vi "WPI_DashboardUpdate Table Values.vi"(11 "Data Values":variant[](array[variant])) -> ()   [LabVIEW 2025]
uses:
  <vilib>/Rock Robotics/WPI/Dashboard/WPI_DashboardLogging Global.vi
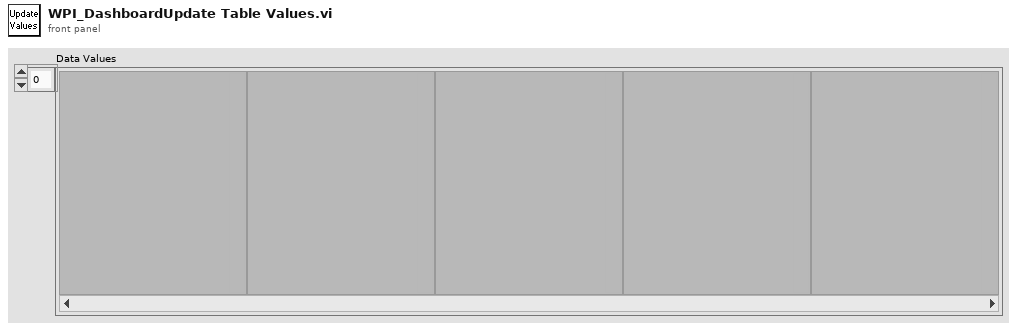
[diagram p1: front panel]
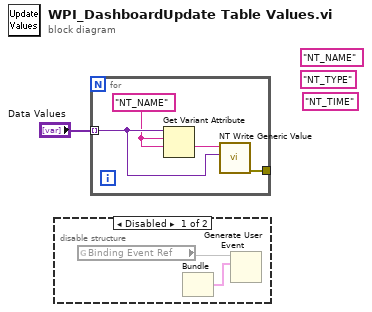
[diagram p0: block diagram]
diagram:
  (unwired) "NT_NAME" ("String")
  (unwired) "NT_TIME" ("String")
  (unwired) "NT_TYPE" ("String")
  n1 = disable-structure shown="Disabled" {
    frame Disabled {
      n2 = global read "WPI_DashboardLogging Global.vi" "Binding Event Ref"() -> (w3)
      n3 = Bundle() -> (w2:cluster{void, void, void})  [unwired: 4 in]
      n4 = Generate User Event(user event=w3, event data cluster=w2) -> ()  [unwired: 2 in, 2 out]
    }
    frame Enabled {
    }
  }
  n5 = for {
    tunnel: "Data Values" -> [w7] mode=indexing
    tunnel: [w4] -> _
    w5 = "NT_NAME" ("String")
    n6 = Get Variant Attribute(Variant=w7, name=w5, default value (empty Variant)=w5) -> (value=w6:string)  [unwired: 1 in, 3 out]
    n7 = call <vilib>:"NT Write Generic Value.vi"("Variant"=w7, "Name"=w6) -> ("error out"=w4:errorcluster)  [unwired: 9 in]
  }
